vi "TL2100LAB04.vi"() -> ()   [LabVIEW 2020]
panel:
  out "System Status":bool
  out "Low Pressure":bool
  out "kPa":dbl(knob) scale=0.0..7.0 scale format="%.0g"
  out "in(H2O)":dbl(knob) scale=0.0..25.0
  out "AtoD":i16 format="%04x"
  out "Volts":dbl(knob) scale=1.0..5.0
  in  "stop":bool
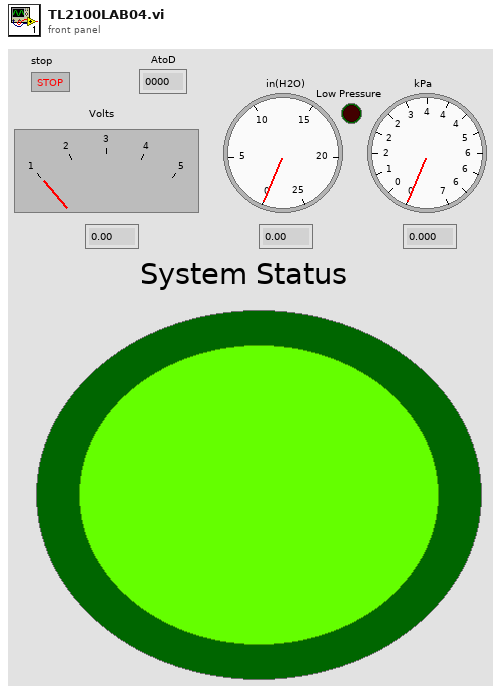
[diagram p1: front panel]
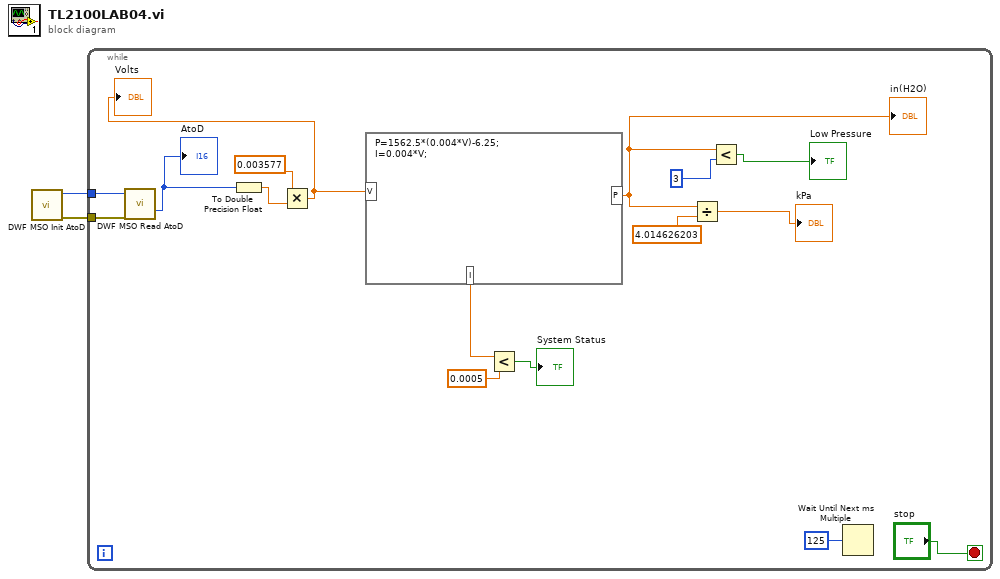
[diagram p0: block diagram]
diagram:
  n1 = call "DWF MSO Init AtoD.vi"() -> ("Error Out"=w1:errorcluster, "Instrument Handle Out"=w2:u32)  [unwired: 10 in]
  n2 = while {
    tunnel: w2 -> [w18]
    tunnel: w1 -> [w17]
    stop <- "stop" stop-if-true
    n3 = call "DWF MSO Read AtoD.vi"("Instrument Handle In AtoD"=w18, "Error In"=w17) -> ("AtoD"=w13:i16)  [unwired: 12 in, 1 out]
    "AtoD" <- w13
    n4 = To Double Precision Float(number=w13) -> (double precision float=w12:dbl)
    n5 = Multiply(x=0.003577, y=w12) -> (x*y=w11:dbl)
    "Volts" <- w11
    n6 = formula code="P=1562.5*(0.004*V)-6.25;\nI=0.004*V;"("V"=w11) -> ("P"=w7:dbl, "I"=w3:dbl)
    "in(H2O)" <- w7
    n7 = Less?(x=w3, y=0.0005) -> (x < y?=→"System Status":bool)
    n8 = Divide(x=w7, y=4.014626203) -> (x/y=→"kPa":dbl)
    n9 = Less?(x=w7, y=3) -> (x < y?=→"Low Pressure":bool)
    n10 = Wait Until Next ms Multiple(millisecond multiple=125) -> ()  [unwired: 1 out]
  }
